vi "Delay.vi"(10 "GF array":dbl[](array[numeric]), 11 "LF array":dbl[](array[numeric])) -> (1 "LF min":dbl, 2 "Delay":i32, 3 "LF max":dbl, 4 "GF min":dbl, 5 "GF max":dbl)   [LabVIEW 2018]
doc: "VI calculates delay w.r.t. grip force and load force peaks."
panel:
  out "max index(es)":i32
  out "GF subarray":dbl[](array[numeric])
  out "LF subarray":dbl[](array[numeric])
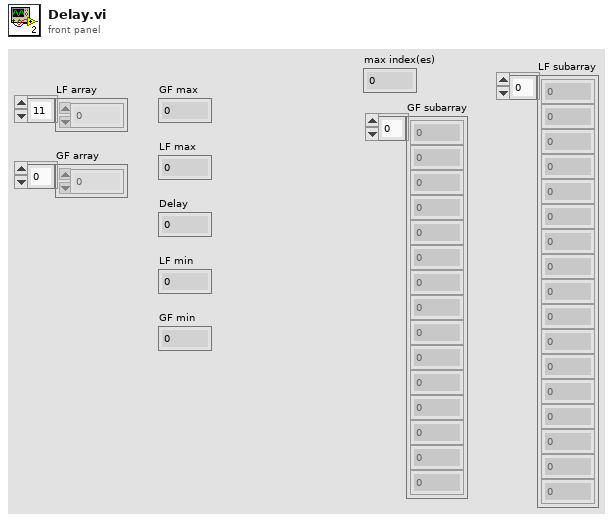
[diagram p1: front panel]
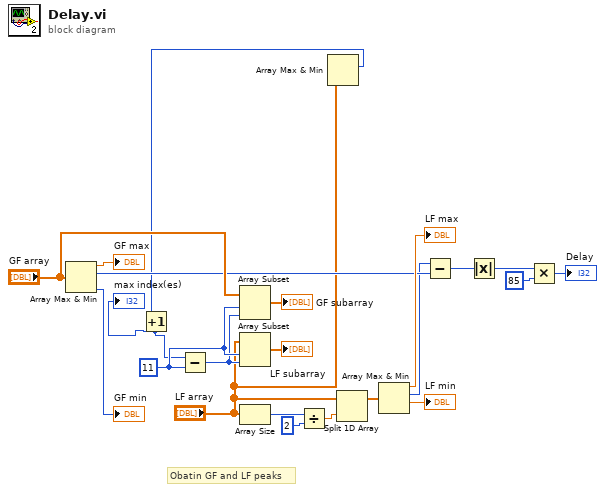
[diagram p0: block diagram]
diagram:
  w8 = 11 ("index")
  # "Obatin GF and LF peaks"
  n1 = Array Max & Min(array="GF array") -> (max value=→"GF max":dbl, max index (indices)=w6:i32, min index (indices)=→"GF min":i32)  [unwired: 1 out]
  n2 = Array Size(array="LF array") -> (size(s)=w20:i32)
  n3 = Divide(x=w20, y=2) -> (x/y=w22:dbl)
  n4 = Array Max & Min(array="LF array") -> (max index (indices)=w2:i32)  [unwired: 3 out]
  n5 = Increment(x=w2) -> (x+1=w1:i32)
  "max index(es)" <- w1
  n6 = Subtract(x=w1, y=w8) -> (x-y=w4:i32)
  n7 = Array Subset(array="GF array", index=w8, length=w4) -> (→"GF subarray":dbl[])
  n8 = Array Subset(array="LF array", index=w8, length=w4) -> (→"LF subarray":dbl[])
  n9 = Split 1D Array(array="LF array", index=w22) -> (first subarray=w11:dbl[])  [unwired: 1 out]
  n10 = Array Max & Min(array=w11) -> (max value=→"LF max":dbl, max index (indices)=w5:i32, min value=→"LF min":dbl)  [unwired: 1 out]
  n11 = Subtract(x=w5, y=w6) -> (x-y=w15:i32)
  n12 = Absolute Value(x=w15) -> (abs(x)=w14:i32)
  n13 = Multiply(x=w14, y=85) -> (x*y=→"Delay":i32)
